vi "1.3.9-Turning Radius.vi"(1 "Wheel Angle":i8) -> (0 "Turning Radius (in)":fxp<+/-,22,12> format="%.14g")   [LabVIEW 2010]
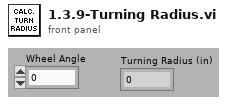
[diagram p1: front panel]
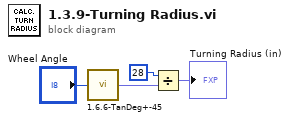
[diagram p0: block diagram]
diagram:
  n1 = call "1.6.6-TanDeg+-45.vi"("theta"="Wheel Angle") -> ("tan(theta)"=w2:fxp<+/-,16,1>)
  n2 = Divide(x=i16 28 ("y"), y=w2) -> (x/y=→"Turning Radius (in)":fxp<+/-,22,12>)
